vi "Shutdown.vi"(8 "error in":errorcluster, 11 "Analog-Output in":refnum<class "Analog-Output.lvclass">) -> (0 "error out":errorcluster, 3 "Analog-Output out":refnum<class "Analog-Output.lvclass">)   [LabVIEW 2019, in "Analog-Output.lvlib" / "Analog-Output.lvclass"]
uses:
  Library/Analog-Output.lvclass
  builds/Instruments/Instruments.lvlibp/Library/Instruments.lvclass
  builds/Engine/Engine.lvlibp/Project/Engine.lvclass
  C:/Users/Public/Documents/Development/builds/Engine/Engine.lvlibp/Project/Engine.lvclass
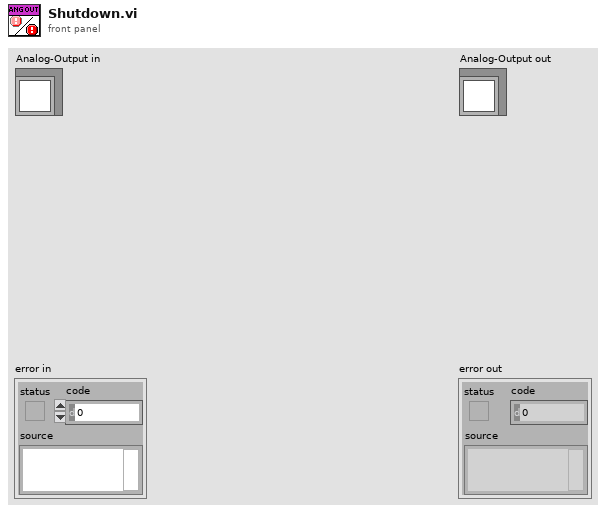
[diagram p1: front panel]
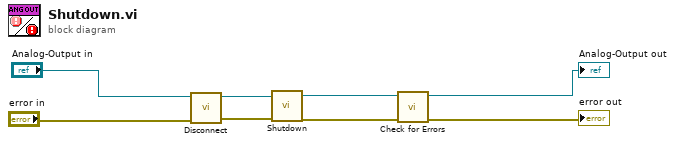
[diagram p0: block diagram]
diagram:
  n1 = call-dynamic "Disconnect.vi"("error in"="error in", "Analog-Output in"="Analog-Output in") -> ("error out"=w7:errorcluster, "Analog-Output out"=w8:refnum<class "Analog-Output.lvclass">)  [unwired: 8 in]
  n2 = call-parent "Shutdown.vi"("error in"=w7, "Instruments in"=w8) -> ("error out"=w3:errorcluster, "Instruments out"=w4:refnum<class "Analog-Output.lvclass">)  [unwired: 8 in]
  n3 = call "Check for Errors.vi"("error in"=w3, "Engine in"=w4) -> ("error out"=→"error out":errorcluster, "Engine out"=→"Analog-Output out":refnum<class "Analog-Output.lvclass">)  [unwired: 8 in]
